vi "send posCov.vi"() -> ()   [LabVIEW 2014]
uses:
  <userlib>/ROS for LabVIEW Software/ROS/Code/Console/Servers/ServerSubs/TopicDef.ctl
  <userlib>/ROS for LabVIEW Software/ROS/Code/SubVIs/_ROSDirection.ctl
  <userlib>/ROS for LabVIEW Software/ROS/Code/_ROSDefinition.vi
  <vilib>/Analysis/7linalg.llb/Create Special Real Matrix.vi
  <vilib>/Analysis/NI_AALPro.lvlib
panel:
  in  "PoseCovariance":T1={"Pose"={"Point"={"x"=0.0, "y"=0.0, "z"=0.0}, "Quaternion"={"x"=0.0, "y"=0.0, "z"=0.0, "w"=0.0}}, "Covariance"=[0.0, 0.0, 0.0, 0.0, 0.0]}
  in  "ROS Master":string="172.16.0.10:11311"
  out "error out":errorcluster
  in  "stop":bool
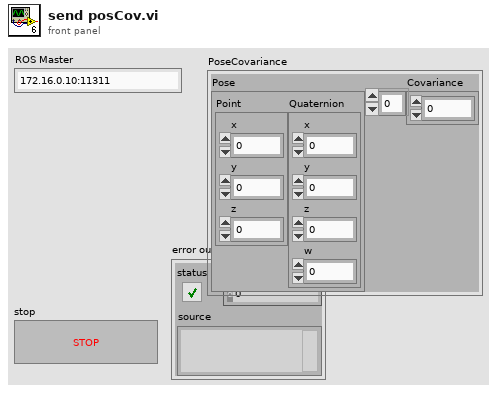
[diagram p1: front panel]
types:
  T1 = cluster{"Pose":cluster{"Point":cluster{"x":dbl, "y":dbl, "z":dbl}, "Quaternion":cluster{"x":dbl, "y":dbl, "z":dbl, "w":dbl}}, "Covariance":dbl[]}
  T2 = typedef "TopicDef.ctl" = cluster{"Topic":string, "Type":string, "Action":T3, "Update (ms)":u16, "queue size":u16}
  T3 = typedef "_ROSDirection.ctl" = enum16{"Node", "Publisher", "Subscriber", "ServiceClient", "ServiceProvider"}
  T4 = typedef "_ROSControl.ctl" = cluster{"topic port":u16, "Node":string, "topic":string, "type":string, "node port":u16, "error ":errorcluster, "Direction":T3, "Update (ms)":u16, "FIFO size":u16}
  T5 = typedef "NI_Matrix.lvlib/RealMatrix.ctl" = dbl[][]
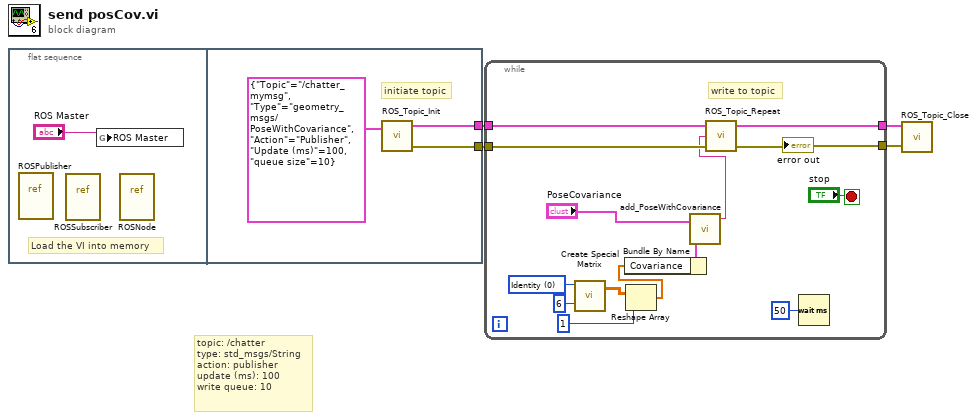
[diagram p0: block diagram]
diagram:
  # "topic: /chatter\ntype: std_msgs/String\naction: publisher\nupdate (ms): 100\nwrite queue: 10"
  n1 = flat-sequence {
    tunnel: [w7] -> w4
    tunnel: [w6] -> w3
    frame #0 {
      # "Load the VI into memory"
      n2 = vi-ref <userlib>:"ROSPublisher.vi"() -> ()  [unwired: 1 out]
      n3 = vi-ref <userlib>:"ROSSubscriber.vi"() -> ()  [unwired: 1 out]
      n4 = global write "_ROSDefinition.vi" "ROS Master"("ROS Master") -> ()
      n5 = vi-ref <userlib>:"ROSNode.vi"() -> ()  [unwired: 1 out]
    }
    frame #1 {
      # "initiate topic"
      n6 = call <userlib>:"ROS_Topic_Init.vi"("Definitions"=T2 {"Topic"="/chatter_mymsg", "Type"="geometry_msgs/PoseWithCovariance", "Action"=enum."Publisher", "Update (ms)"=100, "queue size"=10}) -> ("ROS out"=w7:T4, "error out"=w6:errorcluster)  [unwired: 2 in]
    }
  }
  n7 = while {
    tunnel: w4 -> [w21]
    tunnel: w3 -> [w20]
    tunnel: [w18] -> w2
    tunnel: [w17] -> w1
    stop <- "stop" stop-if-true
    w15 = 0 items=["Identity", "Diagonal", "Toeplitz", "Vandermonde", "Companion", "Hankel", "Hadamard", "Wilkinson", "Hilbert", "Inverse Hilbert", "Rosser", "Pascal"] ("matrix type")
    # "write to topic"
    n8 = call-poly <vilib>:"Create Special Matrix.vi"("matrix type"=w15, "matrix size"=6) -> ("Special Matrix"=w12:T5)  [unwired: 3 in, 1 out]
    n9 = Reshape Array(w12, 1 ("dimension size")) -> (w10:dbl[])
    n10 = Bundle By Name(cluster="PoseCovariance", "Covariance"=w10) -> ()  [unwired: 1 out]
    n11 = call <userlib>:"add_PoseWithCovariance.vi"() -> ("msg out"=w16:string)  [unwired: 5 in]
    n12 = call <userlib>:"ROS_Topic_Repeat.vi"("error in (no error)"=w20, "Msg in"=w16, "ROS in"=w21) -> ("error out"=w17:errorcluster, "ROS out"=w18:T4)  [unwired: 1 in]
    "error out" <- w17
    n13 = Wait (ms)(milliseconds to wait=u32 50) -> ()  [unwired: 1 out]
  }
  n14 = call <userlib>:"ROS_Topic_Close.vi"("error in"=w1, "ROS in"=w2) -> ()  [unwired: 2 in, 1 out]
